vi "To String Helper.vi"(6 "pretty print? (T)":bool=TRUE, 7 "enable LabVIEW extensions? (T)":bool=TRUE, 8 "error in (no error)":errorcluster, 10 "indent":i32, 11 "JSON Value in":refnum<class "JSON Value.lvclass">) -> (0 "error out":errorcluster, 3 "String":string)   [LabVIEW 2016, in "JSON Value.lvclass"]
uses:
  JSON Value.lvclass
  JSON Value.lvclass/JSON Value.ctl
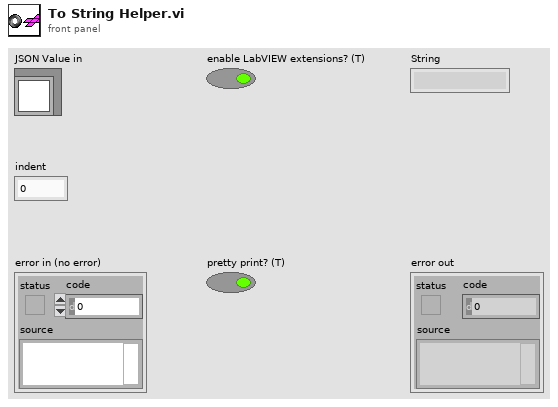
[diagram p1: front panel]
types:
  T1 = typedef "JSON Value.lvclass/JSON Types.ctl" = enum8{"String", "Numeric", "Boolean", "NULL", "Object", "Array"}
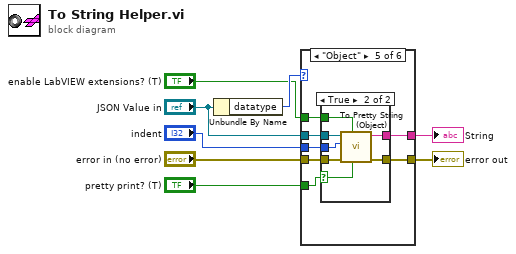
[diagram p0: block diagram]
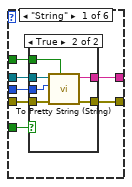
[diagram p2: hidden frame]
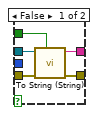
[diagram p3: hidden frame]
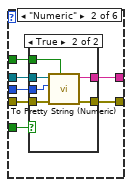
[diagram p4: hidden frame]
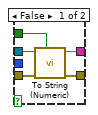
[diagram p5: hidden frame]
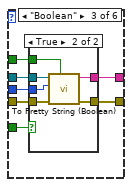
[diagram p6: hidden frame]
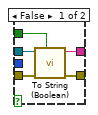
[diagram p7: hidden frame]
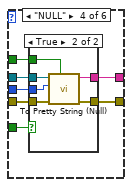
[diagram p8: hidden frame]
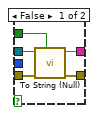
[diagram p9: hidden frame]
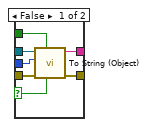
[diagram p10: hidden frame]
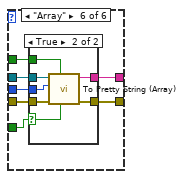
[diagram p11: hidden frame]
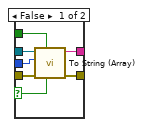
[diagram p12: hidden frame]
diagram:
  n1 = Unbundle By Name("JSON Value in") -> ("datatype"=w8:T1)
  n2 = case shown="\"Object\"" w8 {
    tunnel: [w15 w33 w51 w69 w87 w108] -> w7
    tunnel: [w14 w32 w50 w68 w86 w107] -> w6
    tunnel: "enable LabVIEW extensions? (T)" -> [w13 w31 w49 w67 w85 w106]
    tunnel: "error in (no error)" -> [w12 w30 w48 w66 w84 w105]
    tunnel: "JSON Value in" -> [w11 w29 w47 w65 w83 w104]
    tunnel: "pretty print? (T)" -> [w10 w27 w46 w64 w82 w103]
    tunnel: "indent" -> [w9 w28 w45 w63 w81 w102]
    frame "String" {
      n3 = case shown="True" w10 {
        tunnel: [w20 w26] -> w15
        tunnel: [w19 w23] -> w14
        tunnel: w13 -> [w18 w21]
        tunnel: w12 -> [w17 w25]
        tunnel: w11 -> [w16 w24]
        tunnel: w9 -> [_ w22]
        frame False {
          n4 = call "To String (String).vi"("enable LabVIEW extensions? (T)"=w18, "error in (no error)"=w17, "JSON Value in"=w16) -> ("error out"=w20:errorcluster, "String"=w19:string)  [unwired: 7 in]
        }
        frame True {
          n5 = call "To Pretty String (String).vi"("enable LabVIEW extensions? (T)"=w21, "error in (no error)"=w25, "indent"=w22, "JSON Value in"=w24) -> ("error out"=w26:errorcluster, "String"=w23:string)  [unwired: 6 in]
        }
      }
    }
    frame "Numeric" {
      n6 = case shown="True" w27 {
        tunnel: [w38 w44] -> w33
        tunnel: [w37 w39] -> w32
        tunnel: w31 -> [w36 w40]
        tunnel: w30 -> [w35 w42]
        tunnel: w29 -> [w34 w43]
        tunnel: w28 -> [_ w41]
        frame False {
          n7 = call "To String (Numeric).vi"("enable LabVIEW extensions? (T)"=w36, "error in (no error)"=w35, "JSON Value in"=w34) -> ("error out"=w38:errorcluster, "String"=w37:string)  [unwired: 7 in]
        }
        frame True {
          n8 = call "To Pretty String (Numeric).vi"("enable LabVIEW extensions? (T)"=w40, "error in (no error)"=w42, "indent"=w41, "JSON Value in"=w43) -> ("error out"=w44:errorcluster, "String"=w39:string)  [unwired: 6 in]
        }
      }
    }
    frame "Boolean" {
      n9 = case shown="True" w46 {
        tunnel: [w56 w57] -> w51
        tunnel: [w55 w58] -> w50
        tunnel: w49 -> [w54 w59]
        tunnel: w48 -> [w53 w62]
        tunnel: w47 -> [w52 w61]
        tunnel: w45 -> [_ w60]
        frame False {
          n10 = call "To String (Boolean).vi"("enable LabVIEW extensions? (T)"=w54, "error in (no error)"=w53, "JSON Value in"=w52) -> ("error out"=w56:errorcluster, "String"=w55:string)  [unwired: 7 in]
        }
        frame True {
          n11 = call "To Pretty String (Boolean).vi"("enable LabVIEW extensions? (T)"=w59, "error in (no error)"=w62, "indent"=w60, "JSON Value in"=w61) -> ("error out"=w57:errorcluster, "String"=w58:string)  [unwired: 6 in]
        }
      }
    }
    frame "NULL" {
      n12 = case shown="True" w64 {
        tunnel: [w74 w80] -> w69
        tunnel: [w73 w79] -> w68
        tunnel: w67 -> [w72 w75]
        tunnel: w66 -> [w71 w77]
        tunnel: w65 -> [w70 w78]
        tunnel: w63 -> [_ w76]
        frame False {
          n13 = call "To String (Null).vi"("enable LabVIEW extensions? (T)"=w72, "error in (no error)"=w71, "JSON Datatype in"=w70) -> ("error out"=w74:errorcluster, "String"=w73:string)  [unwired: 7 in]
        }
        frame True {
          n14 = call "To Pretty String (Null).vi"("enable LabVIEW extensions? (T)"=w75, "error in (no error)"=w77, "indent"=w76, "JSON Datatype in"=w78) -> ("error out"=w80:errorcluster, "String"=w79:string)  [unwired: 6 in]
        }
      }
    }
    frame "Object" {
      n15 = case shown="True" w82 {
        selector: w82 -> [w89 w101]
        tunnel: [w94 w97] -> w87
        tunnel: [w93 w99] -> w86
        tunnel: w85 -> [w92 w98]
        tunnel: w84 -> [w91 w96]
        tunnel: w83 -> [w90 w100]
        tunnel: w81 -> [w88 w95]
        frame False {
          n16 = call "To String (Object).vi"("pretty print? (T)"=w89, "enable LabVIEW extensions? (T)"=w92, "error in (no error)"=w91, "indent"=w88, "JSON Value in"=w90) -> ("error out"=w94:errorcluster, "String"=w93:string)  [unwired: 5 in]
        }
        frame True {
          n17 = call "To Pretty String (Object).vi"("pretty print? (T)"=w101, "enable LabVIEW extensions? (T)"=w98, "error in (no error)"=w96, "indent"=w95, "JSON Value in"=w100) -> ("error out"=w97:errorcluster, "Pretty Print String"=w99:string)  [unwired: 5 in]
        }
      }
    }
    frame "Array" {
      n18 = case shown="True" w103 {
        selector: w103 -> [w110 w117]
        tunnel: [w115 w121] -> w108
        tunnel: [w114 w122] -> w107
        tunnel: w106 -> [w113 w118]
        tunnel: w105 -> [w112 w120]
        tunnel: w104 -> [w111 w119]
        tunnel: w102 -> [w109 w116]
        frame False {
          n19 = call "To String (Array).vi"("pretty print? (T)"=w110, "enable LabVIEW extensions? (T)"=w113, "error in (no error)"=w112, "indent"=w109, "JSON Value in"=w111) -> ("error out"=w115:errorcluster, "String"=w114:string)  [unwired: 5 in]
        }
        frame True {
          n20 = call "To Pretty String (Array).vi"("pretty print? (T)"=w117, "enable LabVIEW extensions? (T)"=w118, "error in (no error)"=w120, "indent"=w116, "JSON Value in"=w119) -> ("error out"=w121:errorcluster, "Pretty Print String"=w122:string)  [unwired: 5 in]
        }
      }
    }
  }
  "error out" <- w7
  "String" <- w6
